vi "testWillHeadingHitObstacles.vi"() -> ()   [LabVIEW 2013]
uses:
  Data/TypeDefs/UTM Location.ctl
  Obstacle.lvclass
panel:
  in  "Input List of UTM locations to be arranged into segments":T1[](array[typedef])=[{"UTM Zone"=0.0, "Hemisphere"=enum."North", "East"=0.0, "North"=0.0}, {"UTM Zone"=0.0, "Hemisphere"=enum."North", "East"=5.0, "North"=0.0}, {"UTM Zone"=0.0, "Hemisphere"=enum."North", "East"=0.0, "North"=5.0}, {"UTM Zone"=0.0, "Hemisphere"=enum."North", "East"=-5.0, "North"=0.0}] {"North" format="%#_10f"; "East" format="%#_8f"}
  out "Intersecting obstacles array 2":bool[](array[boolean])
  out "ANY intersecting obstacles?":bool
  in  "Safety offset around edges (m)":dbl=5.0
  in  "Heading":dbl=50.0
  in  "Boat":T1={"UTM Zone"=0.0, "Hemisphere"=enum."North", "East"=0.0, "North"=-5.0} {"North" format="%#_10f"; "East" format="%#_8f"}
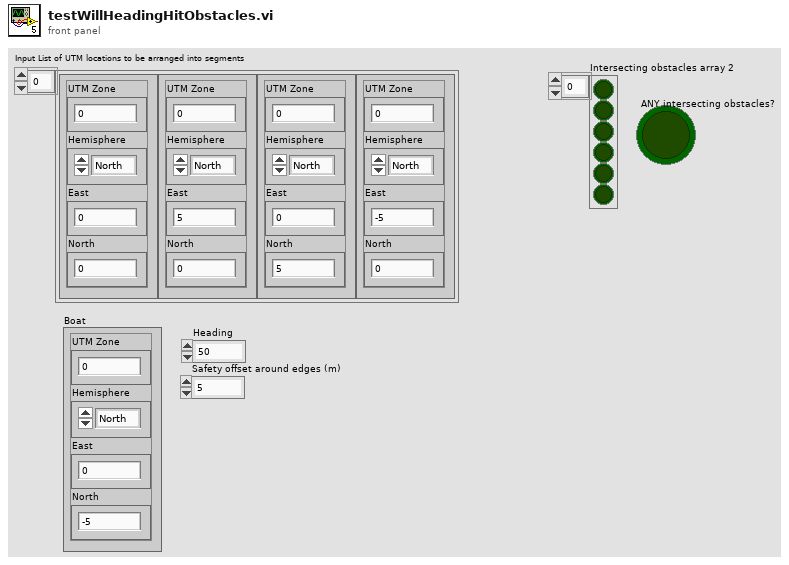
[diagram p1: front panel]
types:
  T1 = typedef "UTM Location.ctl" = cluster{"UTM Zone":dbl, "Hemisphere":enum16{"North", "South"}, "East":dbl, "North":dbl}
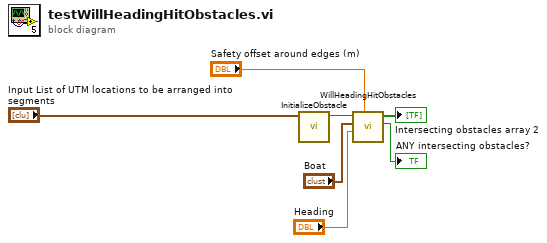
[diagram p0: block diagram]
diagram:
  n1 = call "InitializeObstacle.vi"("Input List of UTM locations to be arranged into segments"="Input List of UTM locations to be arranged into segments") -> ("Obstacle.lvclass"=w7:refnum<class "Obstacle.lvclass">)  [unwired: 10 in]
  n2 = call "WillHeadingHitObstacles.vi"("Safety offset around edges (m)"="Safety offset around edges (m)", "Heading"="Heading", "Boat"="Boat", "Obstacle.lvclass"=w7) -> ("Any intersecting obstacles?"=→"ANY intersecting obstacles?":bool, "Intersecting obstacles array"=→"Intersecting obstacles array 2":bool[])  [unwired: 6 in]
